vi "2D数组垂直镜像[I16].vi"(8 "error in (no error)":errorcluster caption="错误输入（无错误）", 11 "数组":i16[][](array[numeric])) -> (0 "error out":errorcluster caption="错误输出", 3 "垂直镜像":i16[][](array[numeric]))   [LabVIEW 2012]
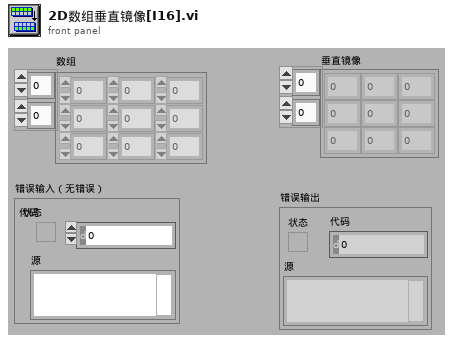
[diagram p1: front panel]
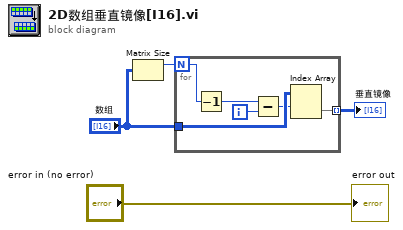
[diagram p0: block diagram]
diagram:
  n1 = Matrix Size(0:"数组") -> (1:w2:i32)  [unwired: 1 out]
  n2 = for {
    N: w2 -> [w10]
    tunnel: "数组" -> [w7]
    tunnel: [w5] -> w1 mode=indexing
    i -> [w8]
    n3 = Decrement(x=w10) -> (x-1=w9:i32)
    n4 = Subtract(x=w9, y=w8) -> (x-y=w6:i32)
    n5 = Index Array(array=w7, index (row)=w6) -> (element=w5:i16[])  [unwired: 1 in]
  }
  "垂直镜像" <- w1
  "error out" <- "error in (no error)"
